vi "ground station.vi"() -> ()   [LabVIEW 2017]
uses:
  C:/Users/Rubidium/source/repos/FABRIK_Solver_CS_FRAME/FABRIK_Solver_CS_FRAME/bin/Debug/FABRIK_Solver_CS_FRAME.dll
  source/repos/FABRIK_Solver_CS_FRAME/FABRIK_Solver_CS_FRAME/bin/Debug/FABRIK_Solver_CS_FRAME.dll
  <vilib>/Analysis/baseanly.llb/A x Vector.vi
  <vilib>/Analysis/NI_AALBase.lvlib
panel:
  in  "局部Z转动":bool
  in  "局部Y转动":bool
  in  "局部X转动":bool
  out "error out":errorcluster
  in  "停止":bool
  in  "目标取向":dbl[][](array[numeric])
  in  "目标位置":dbl[](array[numeric])
  out "求解状态":i32
  out "关节角度":dbl[](array[numeric])
  in  "初始关节位置":dbl[][](array[numeric])
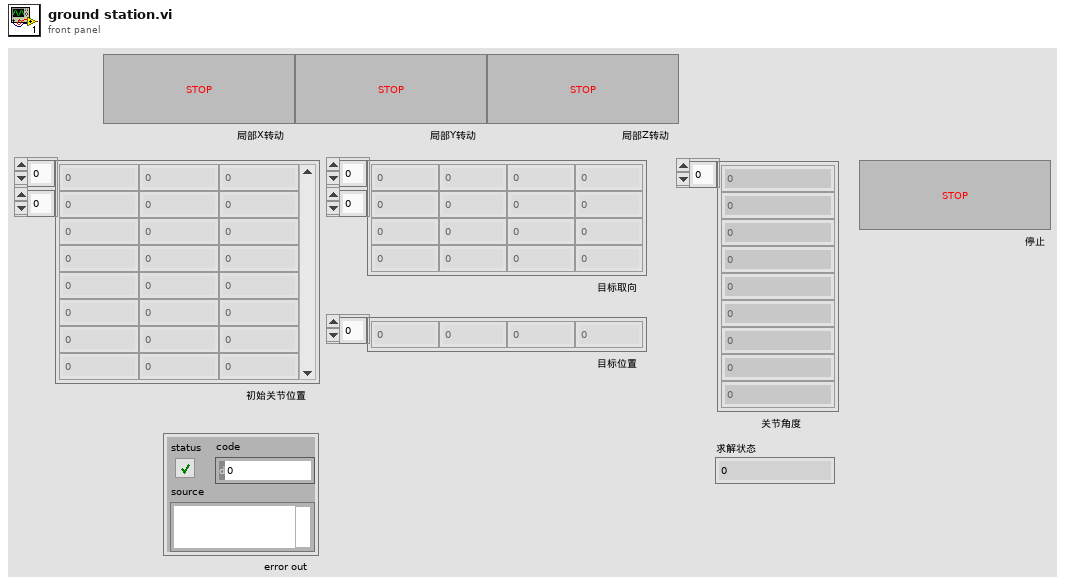
[diagram p1: front panel]
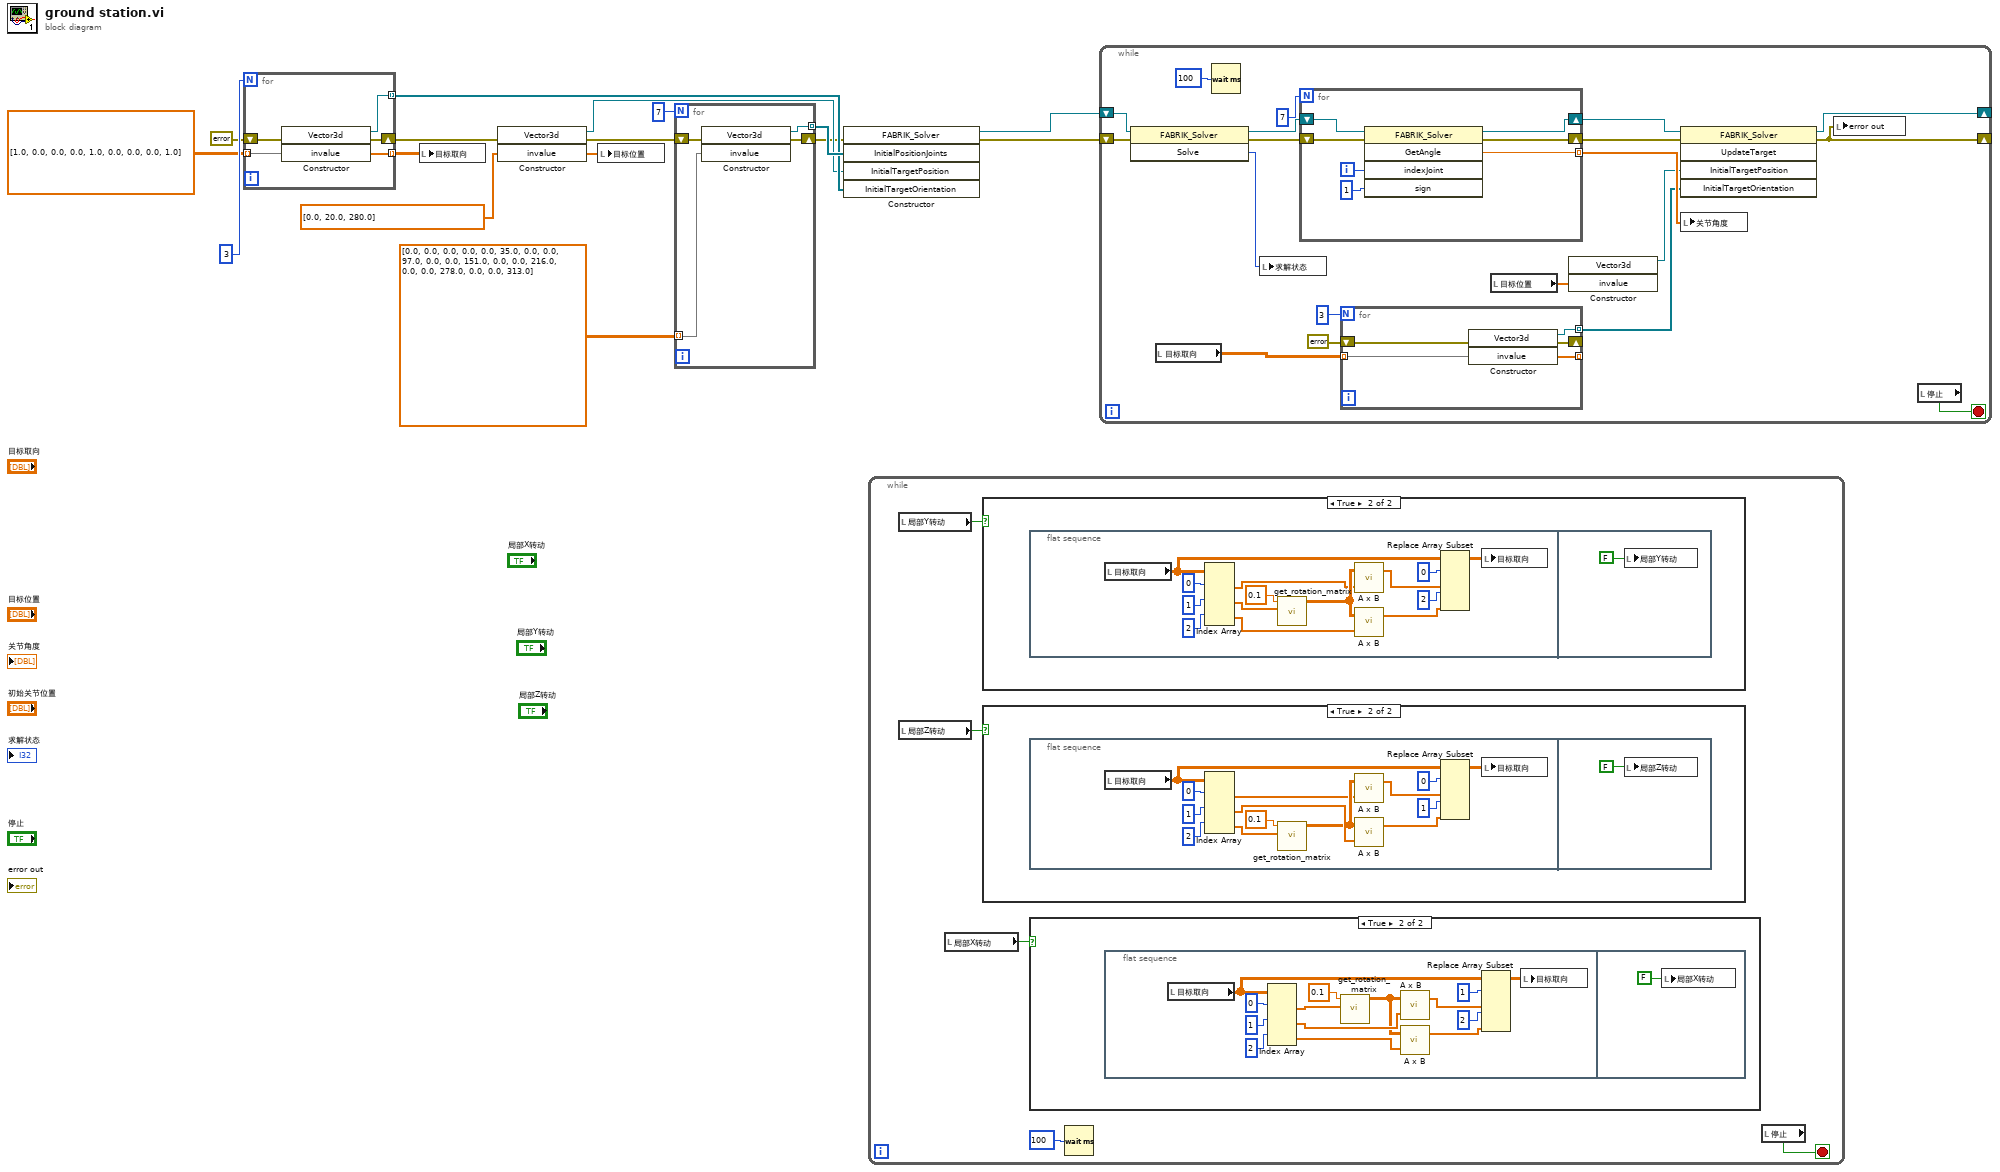
[diagram p0: block diagram]
diagram:
  n1 = for {
    N: 3 -> [_]
    tunnel: dbl[][] [[1.0, 0.0, 0.0], [0.0, 1.0, 0.0], [0.0, 0.0, 1.0]] ("初始关节位置") -> [w21] mode=indexing
    tunnel: [w20] -> w12 mode=indexing
    shift-right: [w18] -> w5
    shift-left: errorcluster {"status"=FALSE, "code"=0, "source"=""} ("error out") -> [w19]
    tunnel: [w17] -> w2 mode=indexing
    n2 = constructor class="Vector3d"(error in=w19, "invalue"=w21) -> (reference out=w20:refnum<k24>, error out=w18:errorcluster, "invalue"=w17:dbl[])  [unwired: 2 in, 1 out]
  }
  n3 = local write "目标取向"(w2) -> ()
  n4 = constructor class="Vector3d"(error in=w5, "invalue"=dbl[] [0.0, 20.0, 280.0] ("初始关节位置")) -> (reference out=w11:refnum<k24>, error out=w4:errorcluster, "invalue"=w1:dbl[])  [unwired: 2 in, 1 out]
  n5 = local write "目标位置"(w1) -> ()
  n6 = for {
    N: 7 -> [_]
    tunnel: dbl[][] [[0.0, 0.0, 0.0], [0.0, 0.0, 35.0], [0.0, 0.0, 97.0], [0.0, 0.0, 151.0], [0.0, 0.0, 216.0], [0.0, 0.0, 278.0], [0.0, 0.0, 313.0]] ("初始关节位置") -> [w22] mode=indexing
    tunnel: [w25] -> w14 mode=indexing
    shift-right: [w24] -> w3
    shift-left: w4 -> [w23]
    n7 = constructor class="Vector3d"(error in=w23, "invalue"=w22) -> (reference out=w25:refnum<k24>, error out=w24:errorcluster)  [unwired: 2 in, 2 out]
  }
  n8 = constructor class="FABRIK_Solver"(error in=w3, "InitialPositionJoints"=w14, "InitialTargetPosition"=w11, "InitialTargetOrientation"=w12) -> (reference out=w16:refnum<k24>, error out=w10:errorcluster)  [unwired: 2 in, 4 out]
  n9 = while {
    stop <- w30 stop-if-true
    n10 = local read "局部Y转动"() -> (w27:bool)
    n11 = local read "局部Z转动"() -> (w26:bool)
    n12 = local read "局部X转动"() -> (w29:bool)
    n13 = case shown="True" w27 {
      frame False {
      }
      frame True {
        n14 = flat-sequence {
          frame #0 {
            n15 = local read "目标取向"() -> (w53:dbl[][])
            n16 = Index Array(array=w53, index (row) #1=0 ("index (row)"), index (row) #2=1 ("index (row)"), index (row) #3=2 ("index (row)")) -> (element #1=w46:dbl[], element #2=w47:dbl[], element #3=w54:dbl[])  [unwired: 3 in]
            n17 = call "get_rotation_matrix.vi"("rotation_axis"=w47, "rotation_angle"=0.1) -> ("rotation_matrix"=w55:dbl[][])  [unwired: 9 in]
            n18 = call-poly <vilib>:"A x B.vi"("Vector"=w46, "A"=w55) -> ("A x Vector"=w50:dbl[])  [unwired: 1 out]
            n19 = call-poly <vilib>:"A x B.vi"("Vector"=w54, "A"=w55) -> ("A x Vector"=w49:dbl[])  [unwired: 1 out]
            n20 = Replace Array Subset(array=w53, new element #1=w50, index (row) #1=0 ("index (row)"), new element #2=w49, index (row) #2=2 ("index (row)")) -> (w48:dbl[][])  [unwired: 2 in]
            n21 = local write "目标取向"(w48) -> ()
          }
          frame #1 {
            n22 = local write "局部Y转动"(FALSE ("局部X转动")) -> ()
          }
        }
      }
    }
    n23 = case shown="True" w26 {
      frame False {
      }
      frame True {
        n24 = flat-sequence {
          frame #0 {
            n25 = local read "目标取向"() -> (w38:dbl[][])
            n26 = Index Array(array=w38, index (row) #1=0 ("index (row)"), index (row) #2=1 ("index (row)"), index (row) #3=2 ("index (row)")) -> (element #1=w33:dbl[], element #2=w40:dbl[], element #3=w34:dbl[])  [unwired: 3 in]
            n27 = call "get_rotation_matrix.vi"("rotation_axis"=w34, "rotation_angle"=0.1) -> ("rotation_matrix"=w39:dbl[][])  [unwired: 9 in]
            n28 = call-poly <vilib>:"A x B.vi"("Vector"=w33, "A"=w39) -> ("A x Vector"=w32:dbl[])  [unwired: 1 out]
            n29 = call-poly <vilib>:"A x B.vi"("Vector"=w40, "A"=w39) -> ("A x Vector"=w31:dbl[])  [unwired: 1 out]
            n30 = Replace Array Subset(array=w38, new element #1=w32, index (row) #1=0 ("index (row)"), new element #2=w31, index (row) #2=1 ("index (row)")) -> (w35:dbl[][])  [unwired: 2 in]
            n31 = local write "目标取向"(w35) -> ()
          }
          frame #1 {
            n32 = local write "局部Z转动"(FALSE ("局部X转动")) -> ()
          }
        }
      }
    }
    n33 = case shown="True" w29 {
      frame False {
      }
      frame True {
        n34 = flat-sequence {
          frame #0 {
            n35 = local read "目标取向"() -> (w66:dbl[][])
            n36 = Index Array(array=w66, index (row) #1=0 ("index (row)"), index (row) #2=1 ("index (row)"), index (row) #3=2 ("index (row)")) -> (element #1=w71:dbl[], element #2=w69:dbl[], element #3=w67:dbl[])  [unwired: 3 in]
            n37 = call "get_rotation_matrix.vi"("rotation_axis"=w71, "rotation_angle"=0.1) -> ("rotation_matrix"=w68:dbl[][])  [unwired: 9 in]
            n38 = call-poly <vilib>:"A x B.vi"("Vector"=w69, "A"=w68) -> ("A x Vector"=w63:dbl[])  [unwired: 1 out]
            n39 = call-poly <vilib>:"A x B.vi"("Vector"=w67, "A"=w68) -> ("A x Vector"=w62:dbl[])  [unwired: 1 out]
            n40 = Replace Array Subset(array=w66, new element #1=w63, index (row) #1=1 ("index (row)"), new element #2=w62, index (row) #2=2 ("index (row)")) -> (w61:dbl[][])  [unwired: 2 in]
            n41 = local write "目标取向"(w61) -> ()
          }
          frame #1 {
            n42 = local write "局部X转动"(FALSE ("局部X转动")) -> ()
          }
        }
      }
    }
    n43 = Wait (ms)(milliseconds to wait=u32 100) -> ()  [unwired: 1 out]
    n44 = local read "停止"() -> (w30:bool)
  }
  n45 = while {
    shift-right: [w87] -> _
    shift-left: w16 -> [w94]
    shift-right: [w77] -> _
    shift-left: w10 -> [w92]
    stop <- w76 stop-if-true
    n46 = invoke class="FABRIK_Solver" method="Solve"(reference=w94, error in=w92) -> (reference out=w91:refnum<k24>, error out=w90:errorcluster, "Solve"=w86:i32)  [unwired: 1 in]
    n47 = local read "目标取向"() -> (w84:dbl[][])
    n48 = Wait (ms)(milliseconds to wait=u32 100) -> ()  [unwired: 1 out]
    n49 = local write "求解状态"(w86) -> ()
    n50 = for {
      N: 7 -> [_]
      tunnel: [w104] -> w89 mode=indexing
      shift-right: [w103] -> w88
      shift-left: w91 -> [w102]
      shift-right: [w100] -> w78
      shift-left: w90 -> [w101]
      i -> [w106]
      n51 = invoke class="FABRIK_Solver" method="GetAngle"(reference=w102, error in=w101, "indexJoint"=w106, "sign"=1) -> (reference out=w103:refnum<k24>, error out=w100:errorcluster, "GetAngle"=w104:dbl)  [unwired: 1 in, 2 out]
    }
    n52 = for {
      N: 3 -> [_]
      tunnel: w84 -> [w99] mode=indexing
      tunnel: [w95] -> w80 mode=indexing
      shift-right: [w97] -> _
      shift-left: errorcluster {"status"=FALSE, "code"=0, "source"=""} ("error out") -> [w98]
      tunnel: [w96] -> _ mode=indexing
      n53 = constructor class="Vector3d"(error in=w98, "invalue"=w99) -> (reference out=w95:refnum<k24>, error out=w97:errorcluster, "invalue"=w96:dbl[])  [unwired: 2 in, 1 out]
    }
    n54 = local read "目标位置"() -> (w82:dbl[])
    n55 = constructor class="Vector3d"("invalue"=w82) -> (reference out=w81:refnum<k24>)  [unwired: 3 in, 3 out]
    n56 = invoke class="FABRIK_Solver" method="UpdateTarget"(reference=w88, error in=w78, "InitialTargetPosition"=w81, "InitialTargetOrientation"=w80) -> (reference out=w87:refnum<k24>, error out=w77:errorcluster)  [unwired: 1 in, 3 out]
    n57 = local write "关节角度"(w89) -> ()
    n58 = local write "error out"(w77) -> ()
    n59 = local read "停止"() -> (w76:bool)
  }
